vi "simple_PID_controller.vi"(6 "Max Integral":dbl, 8 "Reset Integral":bool, 9 "Sensor":dbl, 10 "Setpoint":dbl, 11 "PID Const":T1) -> (3 "Motor Power":dbl)   [LabVIEW 2011]
uses:
  gain_const.ctl
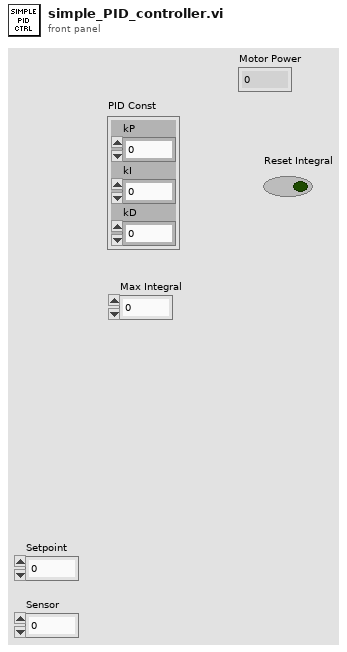
[diagram p1: front panel]
types:
  T1 = typedef "gain_const.ctl" = cluster{"kP":dbl, "kI":dbl, "kD":dbl}
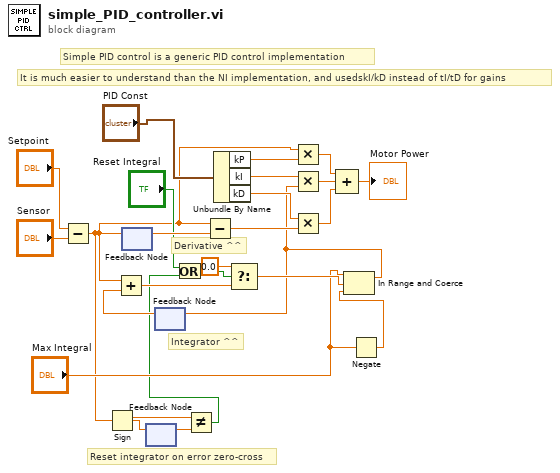
[diagram p0: block diagram]
diagram:
  # "Reset integrator on error zero-cross"
  # "It is much easier to understand than the NI implementation, and usedskI/kD instead of tI/tD for gains"
  # "Simple PID control is a generic PID control implementation"
  # "Derivative ^^"
  # "Integrator ^^"
  n1 = Subtract(x="Setpoint", y="Sensor") -> (x-y=w4:dbl)
  n2 = Sign(1:w4) -> (0:w2:dbl)
  n3 = feedback-in #1(w4) -> ()
  n4 = feedback #1() -> (w15:dbl)  [unwired: 1 in]
  n5 = feedback-in #2(w2) -> ()
  n6 = feedback #2() -> (w1:dbl)  [unwired: 1 in]
  n7 = feedback #3() -> (w20:dbl)  [unwired: 1 in]
  n8 = Add(x=w4, y=w20) -> (x+y=w19:dbl)
  n9 = Not Equal?(x=w2, y=w1) -> (x != y?=w3:bool)
  n10 = Or(x="Reset Integral", y=w3) -> (x .or. y?=w5:bool)
  n11 = Subtract(x=w4, y=w15) -> (x-y=w14:dbl)
  n12 = Unbundle By Name("PID Const") -> ("kP"=w23:dbl, "kI"=w16:dbl, "kD"=w13:dbl)
  n13 = Select(t=0.0, s=w5, f=w19) -> (s? t:f=w10:dbl)
  n14 = Multiply(x=w4, y=w23) -> (x*y=w22:dbl)
  n15 = Multiply(x=w13, y=w14) -> (x*y=w12:dbl)
  n16 = Negate(x="Max Integral") -> (-x=w8:dbl)
  n17 = In Range and Coerce(upper limit="Max Integral", x=w10, lower limit=w8) -> (coerced(x)=w9:dbl)  [unwired: 1 out]
  n18 = feedback-in #3(w9) -> ()
  n19 = Multiply(x=w16, y=w9) -> (x*y=w17:dbl)
  n20 = Compound Arithmetic op=ADD(w22, w17, w12) -> (→"Motor Power":dbl)
